vi "Interpret XY Positions From Raw Data.vi"   [LabVIEW 2013]
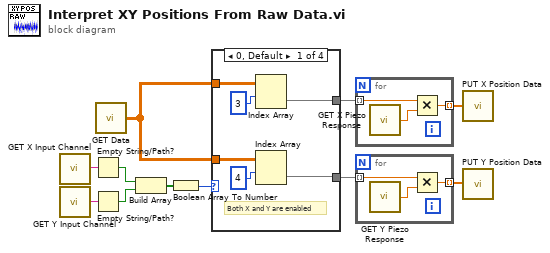
[diagram p0: block diagram]
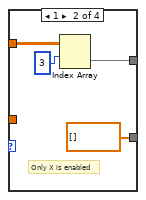
[diagram p2: hidden frame]
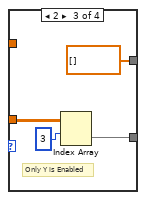
[diagram p3: hidden frame]
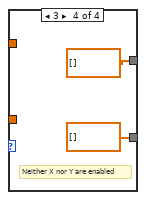
[diagram p4: hidden frame]
diagram:
  n1 = call "GET X Input Channel.vi"() -> ("X Input Channel"=w4:string)
  n2 = call "GET Y Input Channel.vi"() -> ("Y Input Channel"=w3:string)
  n3 = Empty String/Path?(string/path=w4) -> (empty?=w2:bool)
  n4 = Empty String/Path?(string/path=w3) -> (empty?=w5:bool)
  n5 = call "GET Data.vi"() -> ("Data"=w9:dbl[][])
  n6 = Build Array(w2, w5) -> (w1:bool[])
  n7 = Boolean Array To Number(Boolean array=w1) -> (number=w6:u32)
  n8 = case shown="0, Default" w6 {
    tunnel: w9 -> [w16 w20 _ _]
    tunnel: w9 -> [w14 _ w24 _]
    tunnel: [w12 dbl[] [] ("Sensor Data") w23 dbl[] [] ("Sensor Data")] -> w8
    tunnel: [w13 w19 dbl[] [] ("Sensor Data") dbl[] [] ("Sensor Data")] -> w7
    frame 0, Default {
      # "Both X and Y are enabled"
      n9 = Index Array(array=w16, index (row)=3) -> (element=w13:dbl[])  [unwired: 1 in]
      n10 = Index Array(array=w14, index (row)=4) -> (element=w12:dbl[])  [unwired: 1 in]
    }
    frame 1 {
      # "Only X is enabled"
      n11 = Index Array(array=w20, index (row)=3) -> (element=w19:dbl[])  [unwired: 1 in]
    }
    frame 2 {
      # "Only Y is Enabled"
      n12 = Index Array(array=w24, index (row)=3) -> (element=w23:dbl[])  [unwired: 1 in]
    }
    frame 3 {
      # "Neither X nor Y are enabled"
    }
  }
  n13 = for {
    tunnel: w7 -> [w30] mode=indexing
    tunnel: [w28] -> w10 mode=indexing
    n14 = call "GET X Piezo Response.vi"() -> ("X Piezo Response"=w29:dbl)
    n15 = Multiply(x=w30, y=w29) -> (x*y=w28:dbl)
  }
  n16 = for {
    tunnel: w8 -> [w33] mode=indexing
    tunnel: [w31] -> w11 mode=indexing
    n17 = call "GET Y Piezo Response.vi"() -> ("Y Piezo Response"=w32:dbl)
    n18 = Multiply(x=w33, y=w32) -> (x*y=w31:dbl)
  }
  n19 = call "PUT X Position Data.vi"("X Position Data"=w10) -> ()
  n20 = call "PUT Y Position Data.vi"("Y Position Data"=w11) -> ()
